vi "Plot Intermediate Structures.vi"() -> ()   [LabVIEW 2010]
uses:
  <vilib>/picture/3D Picture Control/NI_3D Picture Control.lvlib
panel:
  in  "Boolean":bool
  in  "# Frames 2":i32(slide)=5 scale=0.0..9.0
  out "Atomic Structure":refnum<vi>(3d-picture)
  in  "# Frames":i32(slide)=5 scale=0.0..100.0
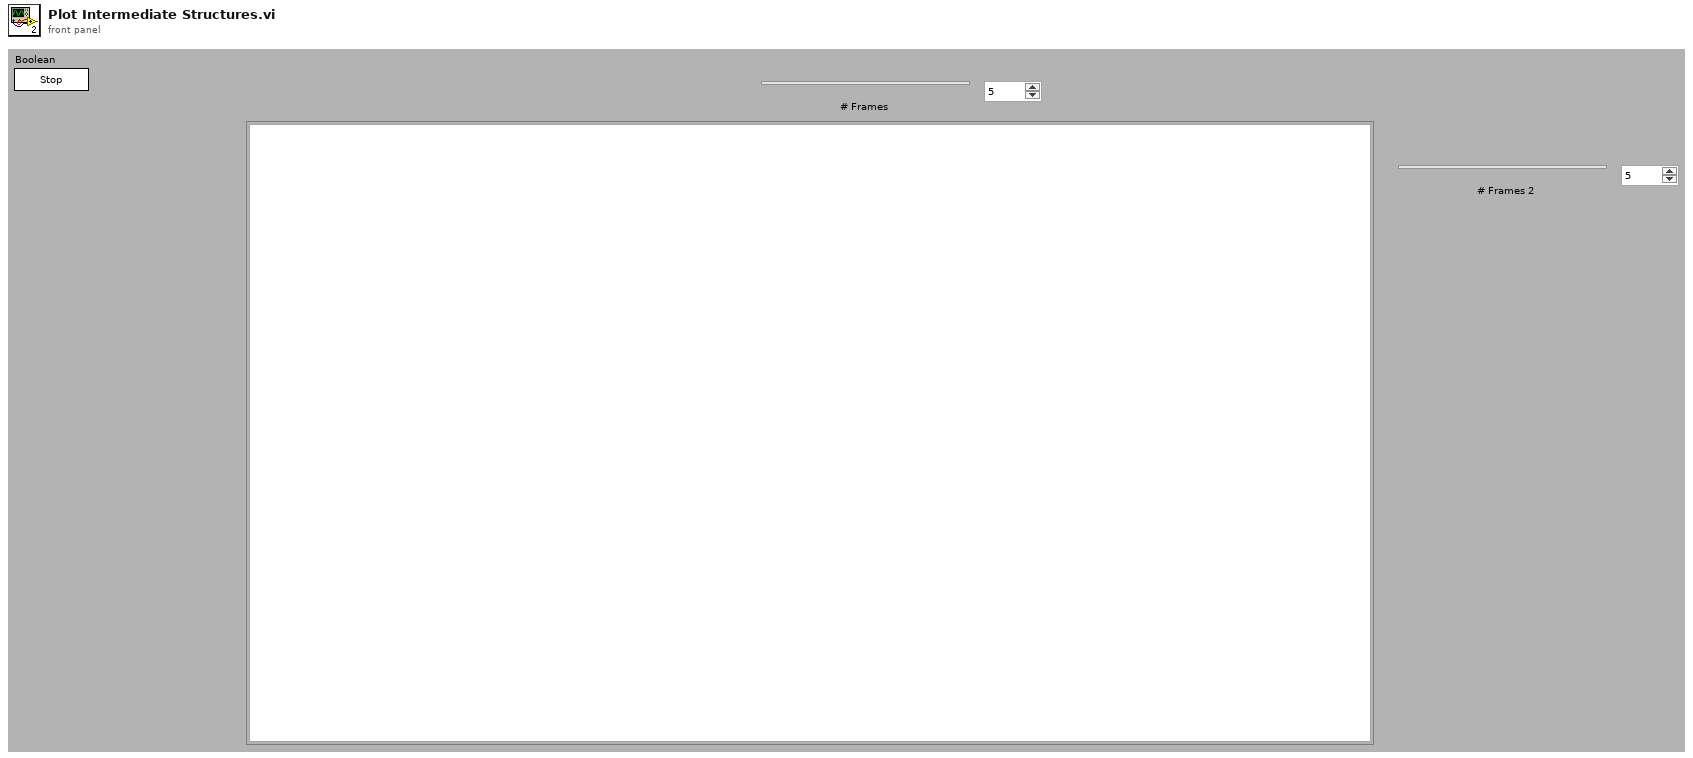
[diagram p1: front panel]
types:
  T1 = cluster{"Structure Name":string, "Lattice vector a":dbl[], "Lattice vector b":dbl[], "Lattice vector c":dbl[], "Atoms Array":cluster{"Atom Name":string, "Positions (Direct)":dbl[][], "Positions (Cartesian)":dbl[][]}[], "# of atoms":i32}
  T2 = cluster{"Structure Name":string, "Lattice vector a":dbl[], "Lattice vector b":dbl[], "Lattice vector c":dbl[], "Atoms Array":cluster{"Atom Name":string, "Positions (Direct)":dbl[][], "Positions (Cartesian)":dbl[][]}[], "# of atoms":i32}[]
  T3 = cluster{"Structure ID":string, "Lattice vector a":dbl[], "Lattice vector b":dbl[], "Lattice vector c":dbl[], "Atoms Array":cluster{"Atom Name":string, "Positions (Direct)":dbl[][], "Positions (Cartesian)":dbl[][]}[], "# of atoms":i32}
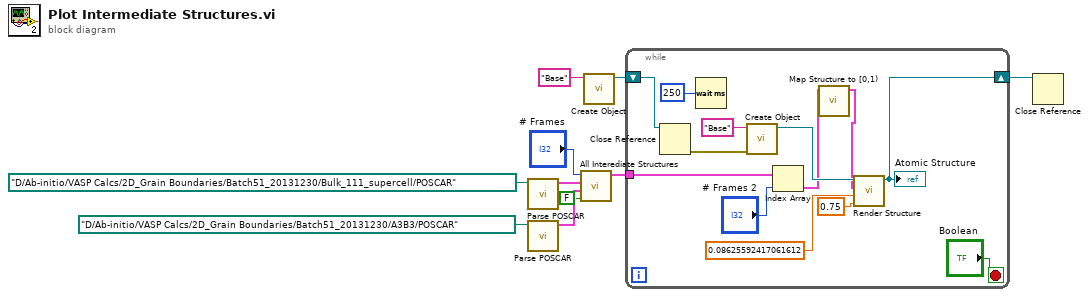
[diagram p0: block diagram]
diagram:
  n1 = call "Parse POSCAR.vi"("POSCAR File"=path "D:/Ab-initio/VASP Calcs/2D_Grain Boundaries/Batch51_20131230/Bulk_111_supercell/POSCAR") -> ("Structure"=w10:T1)  [unwired: 7 in, 3 out]
  n2 = call "Parse POSCAR.vi"("POSCAR File"=path "D:/Ab-initio/VASP Calcs/2D_Grain Boundaries/Batch51_20131230/A3B3/POSCAR") -> ("Structure"=w9:T1)  [unwired: 7 in, 3 out]
  n3 = call "All Interediate Structures.vi"("Map back to [0,1) ?"=FALSE, "Second Structure"=w9, "First Structure"=w10, "# Frames"="# Frames") -> ("Array of Structures"=w4:T2)  [unwired: 7 in]
  n4 = call <vilib>:"Create Object.vi"("Name"="Base") -> ("Scene:New Object"=w3:refnum<vi>)  [unwired: 1 in, 9 out]
  n5 = while {
    tunnel: w4 -> [w23]
    shift-right: [w14] -> w2
    shift-left: w3 -> [w15]
    stop <- "Boolean" stop-if-true
    n6 = Close Reference(reference=w15) -> (error out=w17:errorcluster)  [unwired: 1 in]
    n7 = Wait (ms)(milliseconds to wait=u32 250) -> ()  [unwired: 1 out]
    n8 = call <vilib>:"Create Object.vi"("error in (no error)"=w17, "Name"="Base") -> ("Scene:New Object"=w16:refnum<vi>)  [unwired: 9 out]
    n9 = Index Array(array=w23, index="# Frames 2") -> (element=w12:T1)
    n10 = call "Map Structure to [0,1).vi"("Structure"=w12) -> ("Structure mapped to [0,1)"=w11:T3)  [unwired: 10 in]
    n11 = call "Render Structure.vi"("Atom Size"=0.75, "Scale"=0.08625592417061612, "Atomic Structure"=w11, "Base Object"=w16) -> ("Object with atoms"=w14:refnum<vi>)  [unwired: 7 in]
    "Atomic Structure" <- w14
  }
  n12 = Close Reference(reference=w2) -> ()  [unwired: 1 in, 1 out]
